vi "Msg Post Priority UI Message.vi"(6 "error in (no error)":errorcluster, 7 "Data":variant, 8 "Message":string, 9 "user event":refnum<user-event>) -> (0 "error out":errorcluster, 3 "user event out":refnum<user-event>)   [LabVIEW 2014]
doc: "Post a high priority message to the front of the specified message queue (or event structure). This function does not await a response from the recipient. It is \"fire and forget.\"\n\nThis is part of the Msg suite, intended to make messaging architectures in LabVIEW\nSee the template \"Message Based Application Template.vi\" for normal usage.\n\nCopyright 2005-2016 Jason Sommerville\n\nThis VI may be freely used, modified or distributed under the BSD license."
uses:
  Message Cluster.ctl
  <vilib>/event_ctls.llb/usereventprio.ctl
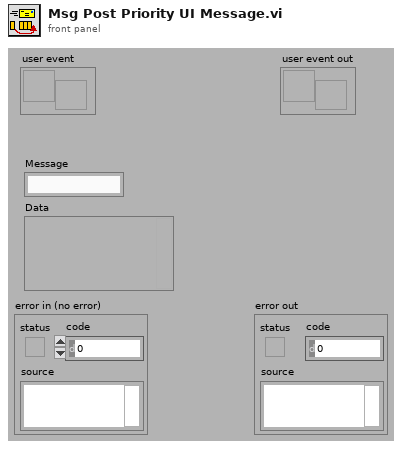
[diagram p1: front panel]
types:
  T1 = typedef "usereventprio.ctl" = enum32{"high priority", "normal priority"}
  T2 = cluster{"Message":string, "Data":variant, refnum<k0>}
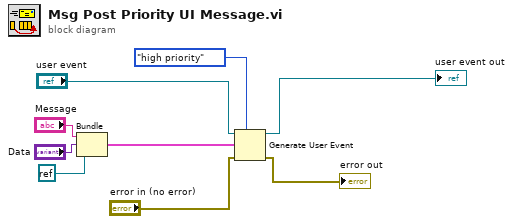
[diagram p0: block diagram]
diagram:
  n1 = Bundle("Message"="Message", "Data"="Data", refnum<k0> refnum) -> (w7:T2)  [unwired: 1 in]
  n2 = Generate User Event(priority (normal)=usereventprio."high priority", user event="user event", event data cluster=w7, error in="error in (no error)") -> (user event out=→"user event out":refnum<user-event>, error out=→"error out":errorcluster)
